vi "Wakeup Message.vi"(8 "error in (no error)":errorcluster, 10 "Wakeup Bit (Set)":cluster{"Address":u16, "Set/Reset":bool}, 11 "Signal Acquisition in":refnum<class "Signal Acquisition.lvclass">) -> (0 "error out":errorcluster, 3 "Signal Acquisition out":refnum<class "Signal Acquisition.lvclass">)   [LabVIEW 2022 SP3, in "Signal Acquisition.lvlib" / "Signal Acquisition.lvclass"]
uses:
  Signal Acquisition.lvclass
  Signal Acquisition.lvclass/Signal Acquisition.ctl
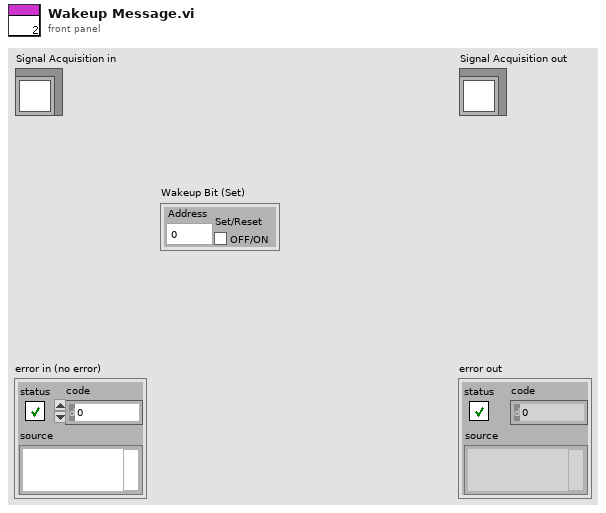
[diagram p1: front panel]
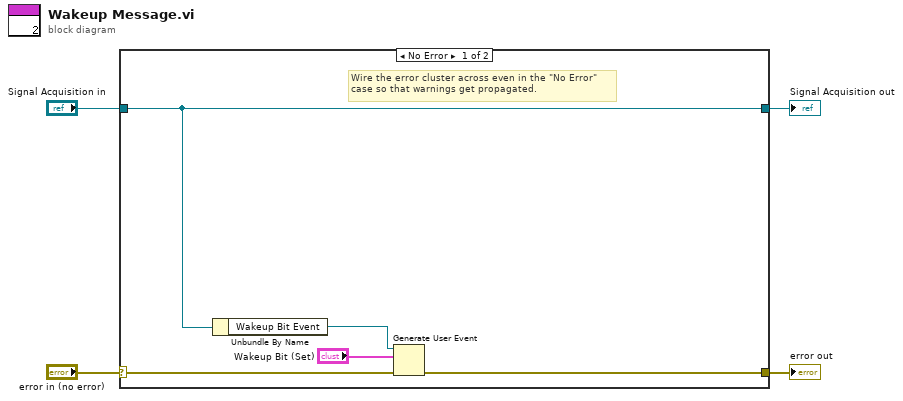
[diagram p0: block diagram]
diagram:
  n1 = case shown="No Error" "error in (no error)" {
    selector: "error in (no error)" -> [w8 w11]
    tunnel: [w7 w11] -> w3
    tunnel: [w9 w10] -> w1
    tunnel: "Signal Acquisition in" -> [w9 w10]
    frame No Error {
      # "Wire the error cluster across even in the \"No Error\"\ncase so that warnings get propagated."
      n2 = Unbundle By Name(w9) -> ("Wakeup Bit Event"=w5:refnum<user-event>)
      n3 = Generate User Event(user event=w5, event data cluster="Wakeup Bit (Set)", error in=w8) -> (error out=w7:errorcluster)  [unwired: 1 in, 1 out]
    }
    frame Error {
    }
  }
  "error out" <- w3
  "Signal Acquisition out" <- w1
